vi "RANGE Header.vi"(4 "Meter 5/6":string, 5 "Meter 3/4":string, 6 "All Meter Data":T1={"Meter 1"={"Meter Size"=0.0, "DAQ Output (Voltage)"=0.0, "Reference (Voltage)"=0.0, "Meter Present"=FALSE, "Meter Visa"="COM3", "Gas Type"="12", "SLPM Error @ Zero"=0.0, "Gas Mix Number"="", "Set STP Register"=FALSE, "Measurement Units"={"Software Rev"="", "Model Number"="", "Manufacturer Info"="", "Software Sub-Rev"="", "Board Rev"="", "Units of Measure Input"={"Abs. Pressure"="", "Gauge/Diff. Press."="", "Barometric Press."="", "Temperature"="", "Volume"="", "Mass"="", "Setpoint"="", "Valve Drive"="", "Totalizer"="", "Tot. Timer"="", "Tot. Avg. Flow"="", "Tot. Peak Flow"=""}}, "Data Frame Format"={"Absolute Pressure"=FALSE, "Gauge/Diff. Pressure"=FALSE, "Barometric Pressure"=FALSE, "Temperature"=FALSE, "Volumetric"=FALSE, "Mass"=FALSE, "Setpoint"=FALSE, "Valve Drive"=FALSE, "Totalizer"=FALSE, "Totalizer Timer"=FALSE, "Totalizer Average Flow"=FALSE, "Totalizer Peak Flow"=FALSE, "Gas Selected"=FALSE, "Tot. Timer Format"=0}}, "Meter 2"={"Meter Size"=0.0, "DAQ Output (Voltage)"=0.0, "Reference (Voltage)"=0.0, "Meter Present"=FALSE, "Meter Visa"="COM3", "Gas Type"="12", "SLPM Error @ Zero"=0.0, "Gas Mix Number"="", "Set STP Register"=FALSE, "Measurement Units"={"Software Rev"="", "Model Number"="", "Manufacturer Info"="", "Software Sub-Rev"="", "Board Rev"="", "Units of Measure Input"={"Abs. Pressure"="", "Gauge/Diff. Press."="", "Barometric Press."="", "Temperature"="", "Volume"="", "Mass"="", "Setpoint"="", "Valve Drive"="", "Totalizer"="", "Tot. Timer"="", "Tot. Avg. Flow"="", "Tot. Peak Flow"=""}}, "Data Frame Format"={"Absolute Pressure"=FALSE, "Gauge/Diff. Pressure"=FALSE, "Barometric Pressure"=FALSE, "Temperature"=FALSE, "Volumetric"=FALSE, "Mass"=FALSE, "Setpoint"=FALSE, "Valve Drive"=FALSE, "Totalizer"=FALSE, "Totalizer Timer"=FALSE, "Totalizer Average Flow"=FALSE, "Totalizer Peak Flow"=FALSE, "Gas Selected"=FALSE, "Tot. Timer Format"=0}}, "Meter 3"={"Meter Size"=0.0, "DAQ Output (Voltage)"=0.0, "Reference (Voltage)"=0.0, "Meter Present"=FALSE, "Meter Visa"="COM3", "Gas Type"="12", "SLPM Error @ Zero"=0.0, "Gas Mix Number"="", "Set STP Register"=FALSE, "Measurement Units"={"Software Rev"="", "Model Number"="", "Manufacturer Info"="", "Software Sub-Rev"="", "Board Rev"="", "Units of Measure Input"={"Abs. Pressure"="", "Gauge/Diff. Press."="", "Barometric Press."="", "Temperature"="", "Volume"="", "Mass"="", "Setpoint"="", "Valve Drive"="", "Totalizer"="", "Tot. Timer"="", "Tot. Avg. Flow"="", "Tot. Peak Flow"=""}}, "Data Frame Format"={"Absolute Pressure"=FALSE, "Gauge/Diff. Pressure"=FALSE, "Barometric Pressure"=FALSE, "Temperature"=FALSE, "Volumetric"=FALSE, "Mass"=FALSE, "Setpoint"=FALSE, "Valve Drive"=FALSE, "Totalizer"=FALSE, "Totalizer Timer"=FALSE, "Totalizer Average Flow"=FALSE, "Totalizer Peak Flow"=FALSE, "Gas Selected"=FALSE, "Tot. Timer Format"=0}}, "Meter 4"={"Meter Size"=0.0, "DAQ Output (Voltage)"=0.0, "Reference (Voltage)"=0.0, "Meter Present"=FALSE, "Meter Visa"="COM3", "Gas Type"="12", "SLPM Error @ Zero"=0.0, "Gas Mix Number"="", "Set STP Register"=FALSE, "Measurement Units"={"Software Rev"="", "Model Number"="", "Manufacturer Info"="", "Software Sub-Rev"="", "Board Rev"="", "Units of Measure Input"={"Abs. Pressure"="", "Gauge/Diff. Press."="", "Barometric Press."="", "Temperature"="", "Volume"="", "Mass"="", "Setpoint"="", "Valve Drive"="", "Totalizer"="", "Tot. Timer"="", "Tot. Avg. Flow"="", "Tot. Peak Flow"=""}}, "Data Frame Format"={"Absolute Pressure"=FALSE, "Gauge/Diff. Pressure"=FALSE, "Barometric Pressure"=FALSE, "Temperature"=FALSE, "Volumetric"=FALSE, "Mass"=FALSE, "Setpoint"=FALSE, "Valve Drive"=FALSE, "Totalizer"=FALSE, "Totalizer Timer"=FALSE, "Totalizer Average Flow"=FALSE, "Totalizer Peak Flow"=FALSE, "Gas Selected"=FALSE, "Tot. Timer Format"=0}}, "Meter 5"={"Meter Size"=0.0, "DAQ Output (Voltage)"=0.0, "Reference (Voltage)"=0.0, "Meter Present"=FALSE, "Meter Visa"="COM3", "Gas Type"="12", "SLPM Error @ Zero"=0.0, "Gas Mix Number"="", "Set STP Register"=FALSE, "Measurement Units"={"Software Rev"="", "Model Number"="", "Manufacturer Info"="", "Software Sub-Rev"="", "Board Rev"="", "Units of Measure Input"={"Abs. Pressure"="", "Gauge/Diff. Press."="", "Barometric Press."="", "Temperature"="", "Volume"="", "Mass"="", "Setpoint"="", "Valve Drive"="", "Totalizer"="", "Tot. Timer"="", "Tot. Avg. Flow"="", "Tot. Peak Flow"=""}}, "Data Frame Format"={"Absolute Pressure"=FALSE, "Gauge/Diff. Pressure"=FALSE, "Barometric Pressure"=FALSE, "Temperature"=FALSE, "Volumetric"=FALSE, "Mass"=FALSE, "Setpoint"=FALSE, "Valve Drive"=FALSE, "Totalizer"=FALSE, "Totalizer Timer"=FALSE, "Totalizer Average Flow"=FALSE, "Totalizer Peak Flow"=FALSE, "Gas Selected"=FALSE, "Tot. Timer Format"=0}}, "Meter 6"={"Meter Size"=0.0, "DAQ Output (Voltage)"=0.0, "Reference (Voltage)"=0.0, "Meter Present"=FALSE, "Meter Visa"="COM3", "Gas Type"="12", "SLPM Error @ Zero"=0.0, "Gas Mix Number"="", "Set STP Register"=FALSE, "Measurement Units"={"Software Rev"="", "Model Number"="", "Manufacturer Info"="", "Software Sub-Rev"="", "Board Rev"="", "Units of Measure Input"={"Abs. Pressure"="", "Gauge/Diff. Press."="", "Barometric Press."="", "Temperature"="", "Volume"="", "Mass"="", "Setpoint"="", "Valve Drive"="", "Totalizer"="", "Tot. Timer"="", "Tot. Avg. Flow"="", "Tot. Peak Flow"=""}}, "Data Frame Format"={"Absolute Pressure"=FALSE, "Gauge/Diff. Pressure"=FALSE, "Barometric Pressure"=FALSE, "Temperature"=FALSE, "Volumetric"=FALSE, "Mass"=FALSE, "Setpoint"=FALSE, "Valve Drive"=FALSE, "Totalizer"=FALSE, "Totalizer Timer"=FALSE, "Totalizer Average Flow"=FALSE, "Totalizer Peak Flow"=FALSE, "Gas Selected"=FALSE, "Tot. Timer Format"=0}}, "Meter Bank 1"={"Flow Rate (BTU/HR)"=0.0, "ANSI Average (BTU/HR)"=0.0, "Panel Data"={"Meter Type (Gas)"="", "Heating Value (BTU/ft³)"=0.0, "Ft³ / Hr (SCFH)"=0.0, "15 Second Average (BTU/HR)"=0.0, "30 Second Average (BTU/HR)"=0.0, "Mass Flow"=0.0, "Vol. Flow"=0.0, "Gas Temperature"=0.0, "Gas Pressure"=0.0, "Tot.Flow"=0.0}, "Meter ID"="", "ANSI Rate"={"ANSI Placeholder Array"=[], "15 Sec Avg Array"=[], "30 Sec Avg Array "=[], "Start ANSI"=FALSE, "ANSI Start Time"=0.0, "Restart ANSI"=FALSE, "ANSI Average (BTU/hr)"=0.0}}, "Meter Bank 2"={"Flow Rate (BTU/HR)"=0.0, "ANSI Average (BTU/HR)"=0.0, "Panel Data"={"Meter Type (Gas)"="", "Heating Value (BTU/ft³)"=0.0, "Ft³ / Hr (SCFH)"=0.0, "15 Second Average (BTU/HR)"=0.0, "30 Second Average (BTU/HR)"=0.0, "Mass Flow"=0.0, "Vol. Flow"=0.0, "Gas Temperature"=0.0, "Gas Pressure"=0.0, "Tot.Flow"=0.0}, "Meter ID"="", "ANSI Rate"={"ANSI Placeholder Array"=[], "15 Sec Avg Array"=[], "30 Sec Avg Array "=[], "Start ANSI"=FALSE, "ANSI Start Time"=0.0, "Restart ANSI"=FALSE, "ANSI Average (BTU/hr)"=0.0}}, "Meter Bank 3"={"Flow Rate (BTU/HR)"=0.0, "ANSI Average (BTU/HR)"=0.0, "Panel Data"={"Meter Type (Gas)"="", "Heating Value (BTU/ft³)"=0.0, "Ft³ / Hr (SCFH)"=0.0, "15 Second Average (BTU/HR)"=0.0, "30 Second Average (BTU/HR)"=0.0, "Mass Flow"=0.0, "Vol. Flow"=0.0, "Gas Temperature"=0.0, "Gas Pressure"=0.0, "Tot.Flow"=0.0}, "Meter ID"="", "ANSI Rate"={"ANSI Placeholder Array"=[], "15 Sec Avg Array"=[], "30 Sec Avg Array "=[], "Start ANSI"=FALSE, "ANSI Start Time"=0.0, "Restart ANSI"=FALSE, "ANSI Average (BTU/hr)"=0.0}}, "Threshold Voltage (NI DAQ)"=0.2, "Use RS232 Data Collection"=FALSE, "Use Auto Switching"=FALSE}, 7 "Meter 1/2":string, 8 "Error In":errorcluster, 9 "Meter Bank 3":bool, 10 "Meter Bank 2":bool, 11 "Meter Bank 1":bool) -> (0 "Error Out":errorcluster, 2 "spreadsheet string":string, 3 "Header":string[](array[string]))   [LabVIEW 2016]
uses:
  Type Definitions/RANGE DAQ Data Four Meters.ctl
  Type Definitions/RANGE DAQ Data.ctl
  Drivers/Omega FMA-1600A Series Gas Flow Meter/Type Definitions/FMA1600A Gas Type.ctl
  Drivers/Omega FMA-1600A Series Gas Flow Meter/Type Definitions/FMA1600A Units String.ctl
  Drivers/Alicat Gas Meter Driver/Sub-VIs/Units of Measure.ctl
  Drivers/Alicat Gas Meter Driver/Sub-VIs/Data Frame.ctl
  Type Definitions/RANGE GAS Data.ctl
  Type Definitions/RANGE Panel Data.ctl
  Type Definitions/RANGE ANSI Rate.ctl
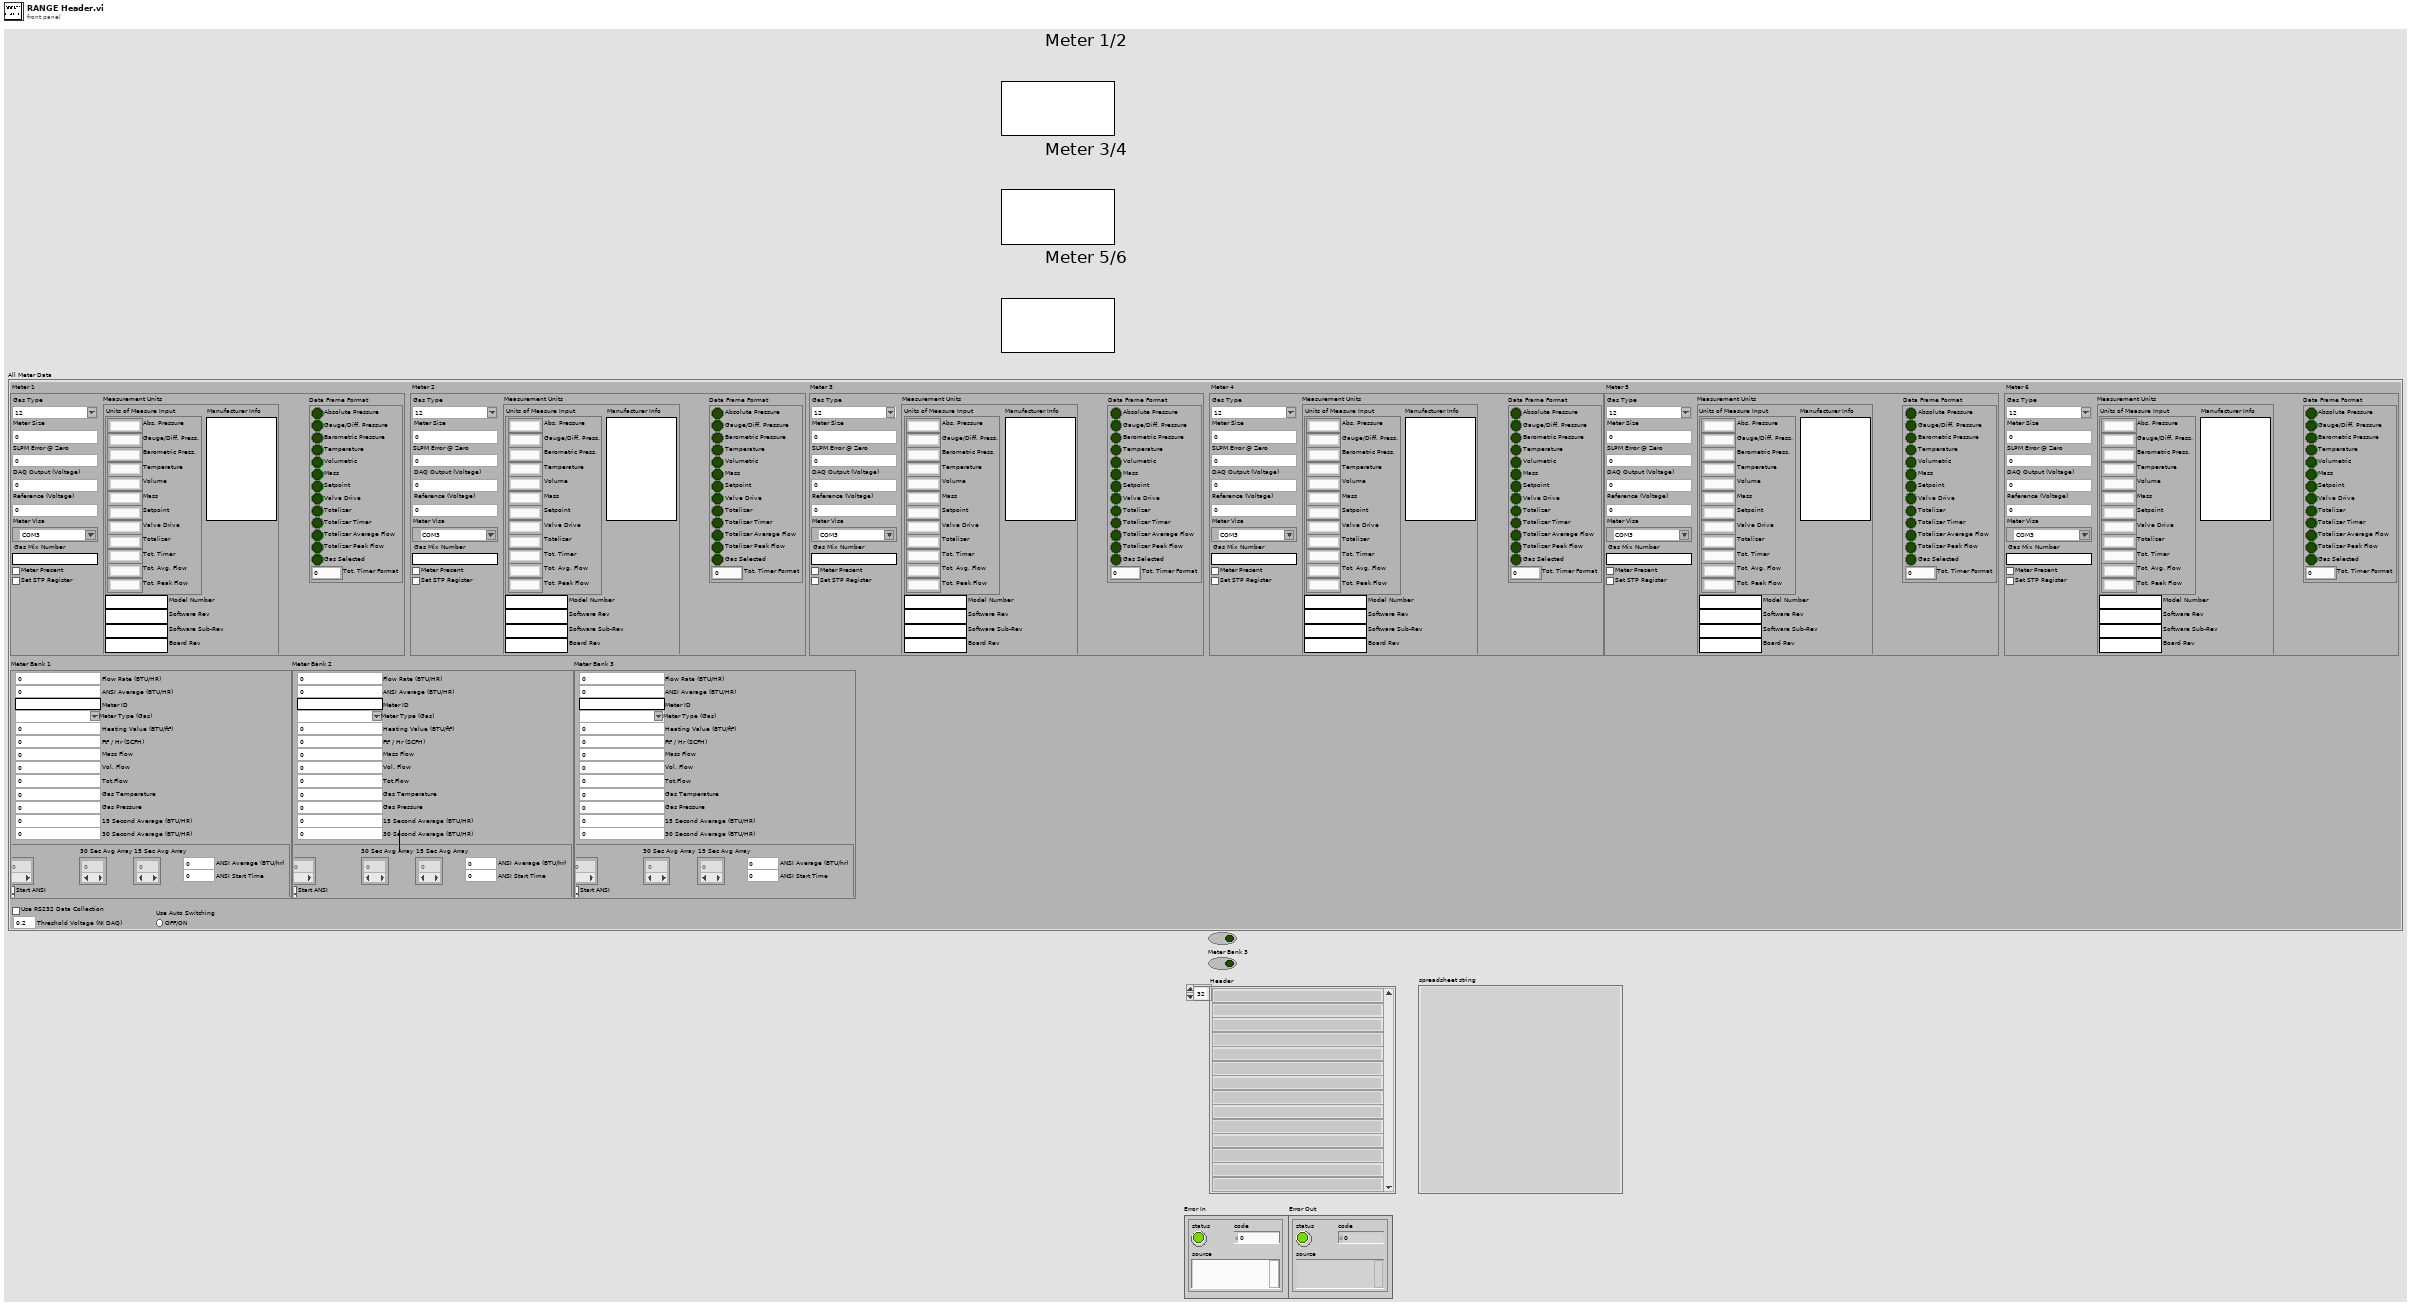
[diagram p1: front panel]
types:
  T1 = typedef "RANGE DAQ Data Four Meters.ctl" = cluster{"Meter 1":T2, "Meter 2":T2, "Meter 3":T2, "Meter 4":T2, "Meter 5":T2, "Meter 6":T2, "Meter Bank 1":T7, "Meter Bank 2":T7, "Meter Bank 3":T7, "Threshold Voltage (NI DAQ)":dbl, "Use RS232 Data Collection":bool, "Use Auto Switching":bool}
  T2 = typedef "RANGE DAQ Data.ctl" = cluster{"Meter Size":dbl, "DAQ Output (Voltage)":dbl, "Reference (Voltage)":dbl, "Meter Present":bool, "Meter Visa":refnum<visa-resource-name>, "Gas Type":T3, "SLPM Error @ Zero":dbl, "Gas Mix Number":string, "Set STP Register":bool, "Measurement Units":T4, "Data Frame Format":T6}
  T3 = typedef "FMA1600A Gas Type.ctl" = string
  T4 = typedef "FMA1600A Units String.ctl" = cluster{"Software Rev":string, "Model Number":string, "Manufacturer Info":string, "Software Sub-Rev":string, "Board Rev":string, "Units of Measure Input":T5}
  T5 = typedef "Units of Measure.ctl" = cluster{"Abs. Pressure":string, "Gauge/Diff. Press.":string, "Barometric Press.":string, "Temperature":string, "Volume":string, "Mass":string, "Setpoint":string, "Valve Drive":string, "Totalizer":string, "Tot. Timer":string, "Tot. Avg. Flow":string, "Tot. Peak Flow":string}
  T6 = typedef "Data Frame.ctl" = cluster{"Absolute Pressure":bool, "Gauge/Diff. Pressure":bool, "Barometric Pressure":bool, "Temperature":bool, "Volumetric":bool, "Mass":bool, "Setpoint":bool, "Valve Drive":bool, "Totalizer":bool, "Totalizer Timer":bool, "Totalizer Average Flow":bool, "Totalizer Peak Flow":bool, "Gas Selected":bool, "Tot. Timer Format":u16}
  T7 = typedef "RANGE GAS Data.ctl" = cluster{"Flow Rate (BTU/HR)":dbl, "ANSI Average (BTU/HR)":dbl, "Panel Data":T8, "Meter ID":string, "ANSI Rate":T9}
  T8 = typedef "RANGE Panel Data.ctl" = cluster{"Meter Type (Gas)":T3, "Heating Value (BTU/ft³)":dbl, "Ft³ / Hr (SCFH)":dbl, "15 Second Average (BTU/HR)":dbl, "30 Second Average (BTU/HR)":dbl, "Mass Flow":dbl, "Vol. Flow":dbl, "Gas Temperature":dbl, "Gas Pressure":dbl, "Tot.Flow":dbl}
  T9 = typedef "RANGE ANSI Rate.ctl" = cluster{"ANSI Placeholder Array":dbl[], "15 Sec Avg Array":dbl[], "30 Sec Avg Array ":dbl[], "Start ANSI":bool, "ANSI Start Time":dbl, "Restart ANSI":bool, "ANSI Average (BTU/hr)":dbl}
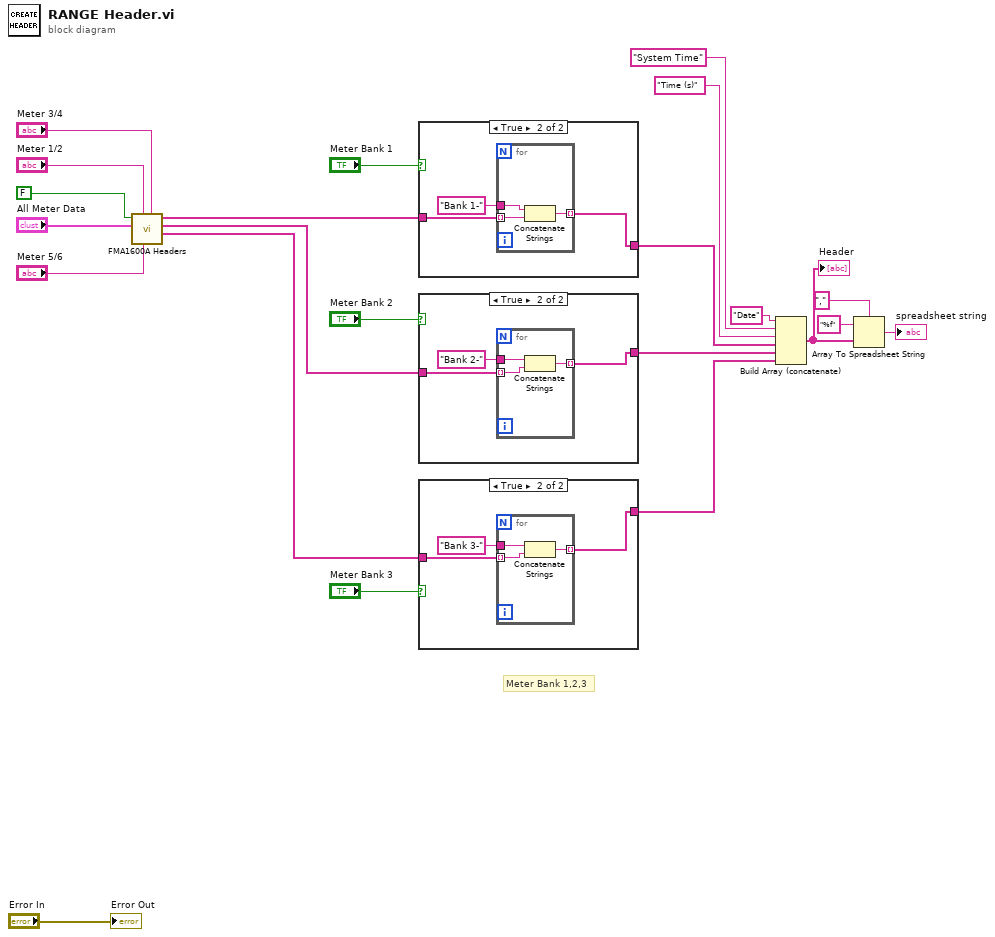
[diagram p0: block diagram]
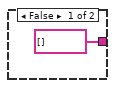
[diagram p2: hidden frame]
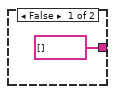
[diagram p3: hidden frame]
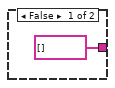
[diagram p4: hidden frame]
diagram:
  # "Meter Bank 1,2,3"
  n1 = call "FMA1600A Headers.vi"("Meter 3/4"="Meter 3/4", "Meter 5/6"="Meter 5/6", "Meter 1/2"="Meter 1/2", "All Meter Data"="All Meter Data", "Dryer?"=FALSE) -> ("Range/Dryer Headers 3"=w4:string[], "Range/Dryer Headers 2"=w5:string[], "Range/Dryer Headers 1"=w11:string[])  [unwired: 3 in, 1 out]
  n2 = case shown="True" "Meter Bank 1" {
    tunnel: [string[] [] w25] -> w14
    tunnel: w11 -> [_ w24]
    frame False {
    }
    frame True {
      n3 = for {
        tunnel: w24 -> [w29] mode=indexing
        tunnel: [w28] -> w25 mode=indexing
        tunnel: "Bank 1-" ("string") -> [w27]
        n4 = Concatenate Strings(w27, w29) -> (w28:string)
      }
    }
  }
  n5 = case shown="True" "Meter Bank 2" {
    tunnel: [string[] [] w32] -> w13
    tunnel: w5 -> [_ w31]
    frame False {
    }
    frame True {
      n6 = for {
        tunnel: w31 -> [w36] mode=indexing
        tunnel: [w35] -> w32 mode=indexing
        tunnel: "Bank 2-" ("string") -> [w34]
        n7 = Concatenate Strings(w34, w36) -> (w35:string)
      }
    }
  }
  n8 = case shown="True" "Meter Bank 3" {
    tunnel: [string[] [] w39] -> w12
    tunnel: w4 -> [_ w38]
    frame False {
    }
    frame True {
      n9 = for {
        tunnel: w38 -> [w43] mode=indexing
        tunnel: [w42] -> w39 mode=indexing
        tunnel: "Bank 3-" ("string") -> [w41]
        n10 = Concatenate Strings(w41, w43) -> (w42:string)
      }
    }
  }
  n11 = Build Array (concatenate)("Date", "System Time", "Time (s)", w14, w13, w12) -> (w18:string[])
  "Header" <- w18
  n12 = Array To Spreadsheet String(delimiter (Tab)=",", array=w18, 3:"%f" ("format string")) -> (spreadsheet string=→"spreadsheet string":string)
  "Error Out" <- "Error In"
